vi "To File (Ref).vi"(0 "refnum in":refnum<file>, 5 "Variant in":variant, 7 "enable LabVIEW extensions? (T)":bool=TRUE, 9 "Pretty Print?":bool=TRUE, 11 "error in (no error)":errorcluster) -> (4 "refnum out":refnum<file>, 15 "error out":errorcluster)   [LabVIEW 2017, in "Advanced Variant Tools.lvlib"]
doc: "Saves a JSON instance's data to the given file."
uses:
  Advanced Variant Tools.lvlib
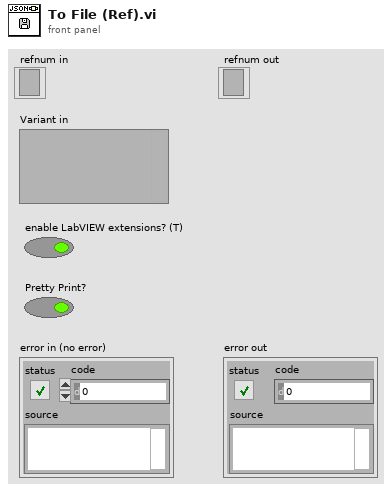
[diagram p1: front panel]
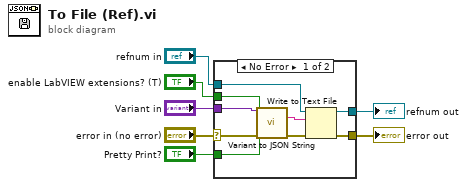
[diagram p0: block diagram]
diagram:
  n1 = case shown="No Error" "error in (no error)" {
    selector: "error in (no error)" -> [w14 w18]
    tunnel: "Variant in" -> [w16 _]
    tunnel: [w11 w18] -> w5
    tunnel: "Pretty Print?" -> [w9 _]
    tunnel: "refnum in" -> [w12 w17]
    tunnel: [w10 w17] -> w2
    tunnel: "enable LabVIEW extensions? (T)" -> [w8 _]
    frame No Error {
      n2 = call "Variant to JSON String.vi"("Variant in"=w16, "enable LabVIEW extensions? (T)"=w8, "pretty print? (F)"=w9, "error in (no error)"=w14) -> ("String"=w15:string, "error out"=w13:errorcluster)  [unwired: 9 in, 1 out]
      n3 = Write to Text File(file (use dialog)=w12, text=w15, error in=w13) -> (refnum out=w10:refnum<file>, error out=w11:errorcluster)  [unwired: 1 in, 1 out]
    }
    frame Error {
    }
  }
  "error out" <- w5
  "refnum out" <- w2
